vi "print.vi"(0 "Standard graph":cluster{"start":sgl, sgl, dbl[][]}(graph)={"start"=190.0, 2.0, []}, 1 "Unknowns graph":cluster{"start":sgl, sgl, dbl[][]}(graph)={"start"=190.0, 2.0, []}, 2 "Sample description":string[](array[string]), 3 "Sample  concentration":dbl[](array[numeric]) format="%.2e", 4 "standard cluster":T3={"Description"="", "Setup"={"integration time"=0.5, "rinse time"=10.0, "sample time"=10.0, "sample type"=0}, "Concentrations"=[], "Absorbance"=[], "Analyst"="", "Concentration units"="", "Good"=[]} {"Absorbance" format="%.2e"; "Concentrations" format="%.2p"; "Setup"."sample type" items=["Sample Cuvet", "Sipper Cell", "No Dialog"]; "Setup"."sample time" min=0.0 max=100.0 step=1.0 format="%.1f"; "Setup"."rinse time" min=0.0 max=100.0 step=1.0 format="%.1f"; "Setup"."integration time" format="%.1f"}, 5 "Sample cluster":T2={"General description"="", "Sample setup"={"integration time"=0.5, "rinse time"=10.0, "sample time"=10.0, "sample type"=0}, "Absorbance"=[], "Analyst"="", "Sample descriptions"=[], "good data"=[]} {"Absorbance" format="%.2e"; "Sample setup"."sample type" items=["Sample Cuvet", "Sipper Cell", "No Dialog"]; "Sample setup"."sample time" min=0.0 max=100.0 step=1.0 format="%.1f"; "Sample setup"."rinse time" min=0.0 max=100.0 step=1.0 format="%.1f"; "Sample setup"."integration time" format="%.1f"}, 11 "Unknown absorbance":dbl[](array[numeric]) format="%.3f", 13 "calibration graph":T4(graph)=[{"Standard"=[], "Standard array"=[]}, {"Standard"=[], "Standard array"=[]}], 15 "slope":dbl format="%.3e", 16 "intercept":dbl format="%.2e", 17 "r":dbl format="%.4f", 18 "wavelength":dbl, 19 "max. conc.":dbl format="%.2e") -> ()   [LabVIEW 2015]
uses:
  settings.ctl
panel:
  in  "ok":bool
  # "Description"
  # "Absorbance"
  # "Concentration"
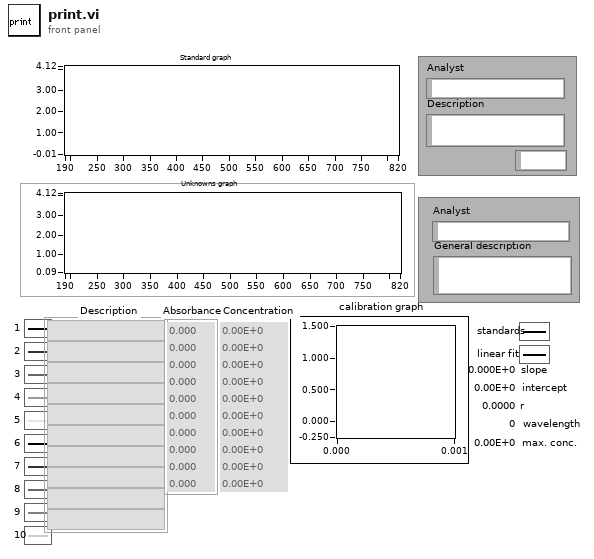
[diagram p1: front panel]
types:
  T1 = typedef "settings.ctl" = cluster{"integration time":sgl, "rinse time":dbl[unit], "sample time":dbl[unit], "sample type":u16}
  T2 = cluster{"General description":string, "Sample setup":T1, "Absorbance":dbl[][], "Analyst":string, "Sample descriptions":string[], "good data":bool[][]}
  T3 = cluster{"Description":string, "Setup":T1, "Concentrations":dbl[], "Absorbance":dbl[][], "Analyst":string, "Concentration units":string, "Good":bool[][]}
  T4 = cluster{"Standard":dbl[], "Standard array":dbl[]}[]
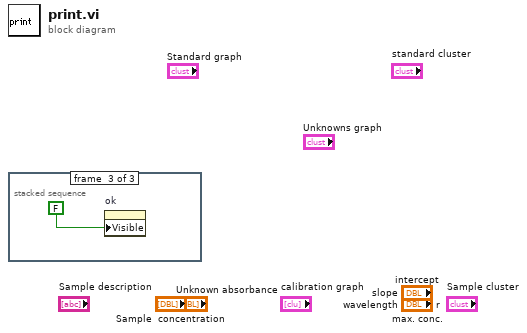
[diagram p0: block diagram]
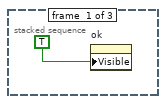
[diagram p2: hidden frame]
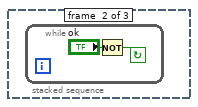
[diagram p3: hidden frame]
diagram:
  n1 = stacked-sequence {
    frame #0 {
      n2 = property on="ok" class="Bool"("Visible"=TRUE) -> ()  [unwired: 2 in, 2 out]
    }
    frame #1 {
      n3 = while {
        stop <- w2 continue-if-true
        n4 = Not(x="ok") -> (.not. x?=w2:bool)
      }
    }
    frame #2 {
      n5 = property on="ok" class="Bool"("Visible"=FALSE) -> ()  [unwired: 2 in, 2 out]
    }
  }
